vi "Set Waiting to Order Queue Handler.vi"(8 "error in (no error)":errorcluster, 10 "Waiting To Order Queue Handler":refnum<class "Job Handler.lvclass">, 11 "Coffee Shop In":refnum<class "Coffee Shop.lvclass">) -> (0 "error out":errorcluster, 3 "Coffee Shop Out":refnum<class "Coffee Shop.lvclass">)   [LabVIEW 2020, in "Coffee Shop.lvclass"]
uses:
  Coffee Shop.lvclass
  C:/Program Files (x86)/National Instruments/LabVIEW 2020/vi.lib/Asteme/Triarc Framework/Process/Process.lvclass
  Process Job/Job Handler.lvclass
  <vilib>/Asteme/Triarc Framework/Process/Process.lvclass/Process.ctl
  <vilib>/Asteme/Triarc Framework/Process/Public/Lifecycle/Get Lifecycle State.vi
  <vilib>/Utility/error.llb/Clear Errors.vi
  <vilib>/Utility/error.llb/Error Cluster From Error Code.vi
  <vilib>/Asteme/Triarc Framework/Process/Process.lvclass
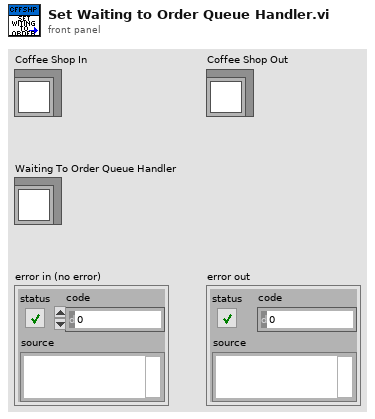
[diagram p1: front panel]
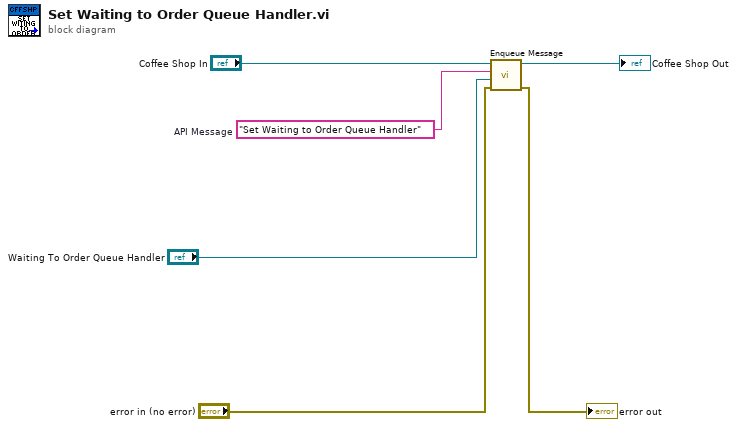
[diagram p0: block diagram]
diagram:
  w3 = "Set Waiting to Order Queue Handler"  # API Message
  n1 = call <vilib>:"Enqueue Message.vi"("error in (no error)"="error in (no error)", "Message Data"="Waiting To Order Queue Handler", "Message"=w3, "Process In"="Coffee Shop In") -> ("error out"=→"error out":errorcluster, "Process Out"=→"Coffee Shop Out":refnum<class "Coffee Shop.lvclass">)  [unwired: 6 in]
